vi "VI Tree.vi"   [LabVIEW 2012, in "Phidget Voltage Input.lvlib"]
doc: "${VoltageInput:VITreeHeader}"
uses:
  <instrlib>/Phidgets/Phidget Voltage Input/Phidget Voltage Input.lvlib
  <instrlib>/Phidgets/Phidget Voltage Input/Public/VoltageInputStart.vi
  <instrlib>/Phidgets/Phidget Voltage Input/Public/VoltageInputOpen.vi
  <instrlib>/Phidgets/Phidget Voltage Input/Public/VoltageInputClose.vi
panel:
  # "(c) 2015 Phidgets Inc..  ALL RIGHTS RESERVED."
  # "SEE DIAGRAM\nFOR VI TREE."
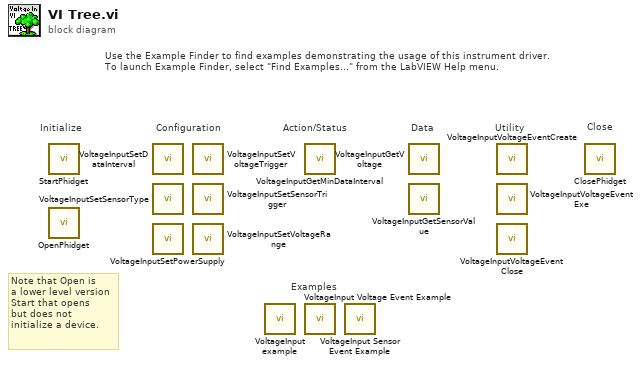
[diagram p0: block diagram]
diagram:
  # "Note that Open is\na lower level version\nStart that opens\nbut does not \ninitialize a device."
  # "Examples"
  # "Use the Example Finder to find examples demonstrating the usage of this instrument driver.\nTo launch Example Finder, select \"Find Examples...\" from the LabVIEW Help menu."
  # "Configuration"
  # "Utility"
  # "Data"
  # "Action/Status"
  # "Close"
  # "Initialize"
  n1 = call-poly <instrlib>:"StartPhidget.vi"() -> ()  [unwired: 12 in, 4 out]
  n2 = call-poly <instrlib>:"OpenPhidget.vi"() -> ()  [unwired: 8 in, 4 out]
  n3 = call <instrlib>:"VoltageInputSetDataInterval.vi"() -> ()  [unwired: 9 in, 2 out]
  n4 = call <instrlib>:"VoltageInputSetSensorType.vi"() -> ()  [unwired: 9 in, 2 out]
  n5 = call <instrlib>:"VoltageInputSetPowerSupply.vi"() -> ()  [unwired: 9 in, 2 out]
  n6 = call <instrlib>:"VoltageInputSetVoltageTrigger.vi"() -> ()  [unwired: 9 in, 2 out]
  n7 = call <instrlib>:"VoltageInputSetSensorTrigger.vi"() -> ()  [unwired: 9 in, 2 out]
  n8 = call <instrlib>:"VoltageInputSetVoltageRange.vi"() -> ()  [unwired: 9 in, 2 out]
  n9 = call <instrlib>:"VoltageInput example.vi"() -> ()  [unwired: 12 in]
  n10 = call <instrlib>:"VoltageInputGetMinDataInterval.vi"() -> ()  [unwired: 8 in, 3 out]
  n11 = call <instrlib>:"VoltageInput Voltage Event Example.vi"() -> ()  [unwired: 12 in]
  n12 = call <instrlib>:"VoltageInput Sensor Event Example.vi"() -> ()  [unwired: 12 in]
  n13 = call <instrlib>:"VoltageInputGetVoltage.vi"() -> ()  [unwired: 8 in, 3 out]
  n14 = call <instrlib>:"VoltageInputGetSensorValue.vi"() -> ()  [unwired: 8 in, 3 out]
  n15 = call <instrlib>:"VoltageInputVoltageEventCreate.vi"() -> ()  [unwired: 9 in, 3 out]
  n16 = call <instrlib>:"VoltageInputVoltageEventExe.vi"() -> ()  [unwired: 5 in, 7 out]
  n17 = call <instrlib>:"VoltageInputVoltageEventClose.vi"() -> ()  [unwired: 10 in, 2 out]
  n18 = call-poly <instrlib>:"ClosePhidget.vi"() -> ()  [unwired: 11 in, 1 out]
